vi "Wait on Token.vi"(1 "Timeout in ms (-1)":i32=-1, 3 "Sync Token Refnum":T1) -> (0 "Timed out?":bool)   [LabVIEW 2019, in "Sync Token.lvlib"]
doc: "Waits for a <b>Sync Token</b> to be signalled using <b>Set Token.vi</b>. This VI blocks execution until the token is set, the specified timeout elapses, or an error occurs."
uses:
  Sync Token.lvlib
  Controls/Public/Sync Token Refnum.ctl
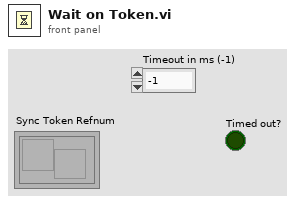
[diagram p1: front panel]
types:
  T1 = typedef "Sync Token.lvlib/Sync Token Refnum.ctl" = refnum<k1>
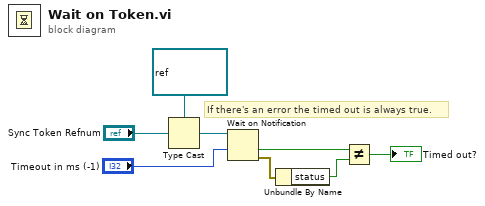
[diagram p0: block diagram]
diagram:
  # "If there's an error the timed out is always true."
  n1 = Type Cast(type=refnum<notifier> refnum ("notifier out"), x="Sync Token Refnum") -> (*(type *) &x=w6:refnum<notifier>)
  n2 = Wait on Notification(notifier=w6, timeout in ms (-1)="Timeout in ms (-1)") -> (timed out?=w3:bool, error out=w5:errorcluster)  [unwired: 2 in, 2 out]
  n3 = Unbundle By Name(w5) -> ("status"=w4:bool)
  n4 = Not Equal?(x=w3, y=w4) -> (x != y?=→"Timed out?":bool)
